vi "List VIs.vi"(8 "error in (no error)":errorcluster, 11 "Rename in":refnum<class "ProjectItem.lvclass">) -> (0 "error out":errorcluster, 3 "Rename out":refnum<class "ProjectItem.lvclass">)   [LabVIEW 2019, in "ProjectItem.lvclass"]
uses:
  ProjectItem.lvclass
  ProjectItem.lvclass/ProjectItem.ctl
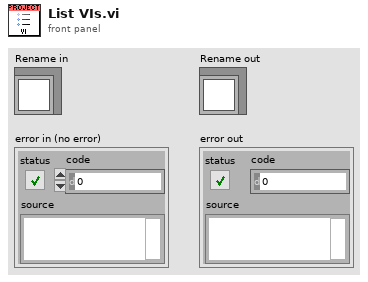
[diagram p1: front panel]
types:
  T1 = cluster{"Class":refnum<vi>, "DynamicVIs":refnum<vi>[], "StaticVIs":refnum<vi>[]}[]
  T2 = cluster{"Class":refnum<vi>, "DynamicVIs":refnum<vi>[], "StaticVIs":refnum<vi>[]}
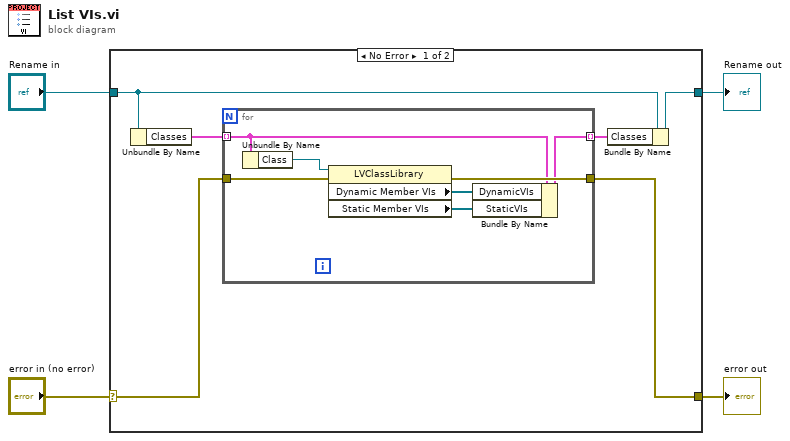
[diagram p0: block diagram]
diagram:
  n1 = case shown="No Error" "error in (no error)" {
    selector: "error in (no error)" -> [w6 w19]
    tunnel: [w9 w18] -> w4
    tunnel: "Rename in" -> [w8 w18]
    tunnel: [w5 w19] -> w2
    frame No Error {
      n2 = Unbundle By Name(w8) -> ("Classes"=w7:T1)
      n3 = for {
        tunnel: w7 -> [w14] mode=indexing
        tunnel: w6 -> [w17]
        tunnel: [w16] -> w5
        tunnel: [w13] -> w10 mode=indexing
        n4 = Unbundle By Name(w14) -> ("Class"=w15:refnum<vi>)
        n5 = property class="LVClassLibrary"(reference=w15, error in=w17) -> (error out=w16:errorcluster, "Dynamic Member VIs"=w12:refnum<vi>[], "Static Member VIs"=w11:refnum<vi>[])  [unwired: 1 out]
        n6 = Bundle By Name(cluster=w14, "DynamicVIs"=w12, "StaticVIs"=w11) -> (w13:T2)
      }
      n7 = Bundle By Name(cluster=w8, "Classes"=w10) -> (w9:refnum<class "ProjectItem.lvclass">)
    }
    frame Error {
    }
  }
  "Rename out" <- w4
  "error out" <- w2
